vi "Winkel Task Starten.vi"(8 "error IO":errorcluster, 11 "Pendelaufbau in":T1(ring)) -> (0 "error out":errorcluster, 2 "Winkel Task":T2)   [LabVIEW 2014]
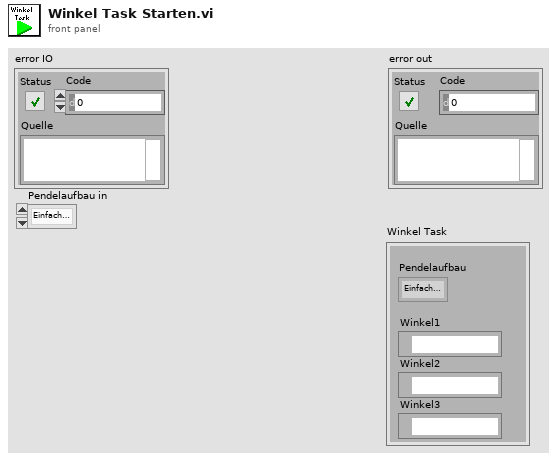
[diagram p1: front panel]
types:
  T1 = enum16{"Einfachpendel", "Doppelpendel", "Dreifachpendel"}
  T2 = cluster{"Pendelaufbau":enum16{"Einfachpendel", "Doppelpendel", "Dreifachpendel"}, "Winkel1":refnum<k21>, "Winkel2":refnum<k21>, "Winkel3":refnum<k21>}
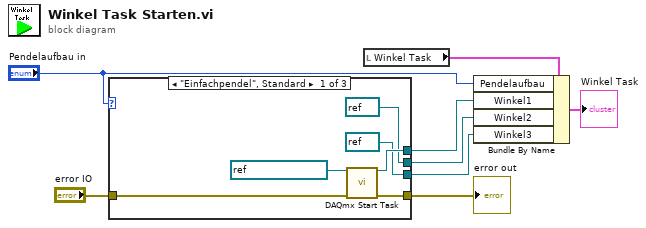
[diagram p0: block diagram]
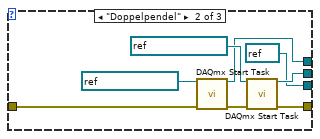
[diagram p2: hidden frame]
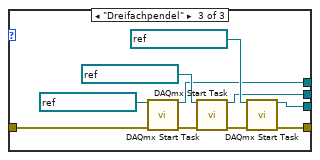
[diagram p3: hidden frame]
diagram:
  n1 = case shown="\"Einfachpendel\", Standard" "Pendelaufbau in" {
    tunnel: "error IO" -> [w14 w19 w27]
    tunnel: [w13 w18 w23] -> w4
    tunnel: [refnum<k21> refnum ("task out") refnum<k21> refnum ("task out") w29] -> w2
    tunnel: [refnum<k21> refnum ("task out") w17 w28] -> w3
    tunnel: [w9 w16 w24] -> w7
    frame "Einfachpendel", Default {
      n2 = call <vilib>:"DAQmx Start Task.vi"("task/channels in"=refnum<k21> "Winkel1 Task", "error in"=w14) -> ("task out"=w13:refnum<k21>, "error out"=w9:errorcluster)  [unwired: 12 in]
    }
    frame "Doppelpendel" {
      n3 = call <vilib>:"DAQmx Start Task.vi"("task/channels in"=refnum<k21> "Winkel1 Task", "error in"=w19) -> ("task out"=w18:refnum<k21>, "error out"=w22:errorcluster)  [unwired: 12 in]
      n4 = call <vilib>:"DAQmx Start Task.vi"("task/channels in"=refnum<k21> "Winkel2 Task", "error in"=w22) -> ("task out"=w17:refnum<k21>, "error out"=w16:errorcluster)  [unwired: 12 in]
    }
    frame "Dreifachpendel" {
      n5 = call <vilib>:"DAQmx Start Task.vi"("task/channels in"=refnum<k21> "Winkel1 Task", "error in"=w27) -> ("task out"=w23:refnum<k21>, "error out"=w26:errorcluster)  [unwired: 12 in]
      n6 = call <vilib>:"DAQmx Start Task.vi"("task/channels in"=refnum<k21> "Winkel2 Task", "error in"=w26) -> ("task out"=w28:refnum<k21>, "error out"=w25:errorcluster)  [unwired: 12 in]
      n7 = call <vilib>:"DAQmx Start Task.vi"("task/channels in"=refnum<k21> "Winkel3 Task", "error in"=w25) -> ("task out"=w29:refnum<k21>, "error out"=w24:errorcluster)  [unwired: 12 in]
    }
  }
  "error out" <- w7
  n8 = local read "Winkel Task"() -> (w5:T2)
  n9 = Bundle By Name(cluster=w5, "Pendelaufbau"="Pendelaufbau in", "Winkel1"=w4, "Winkel2"=w3, "Winkel3"=w2) -> (→"Winkel Task":T2)
